vi "S4GUI_002.vi"(7 "Tab ObsEng":enum32{"Obs", "CCD modes", "Eng"}(tab)) -> ()   [LabVIEW 2018] (continued)
            n4169 = call-dynamic "Write Cooler ON_OFF.vi"("error in (no error)"=w9735, "Cooler ON/OFF"=w9727, "Interface in"=w9736) -> ("error out"=w9739:errorcluster, "Interface out"=w9741:refnum<class "Interface.lvclass">)  [unwired: 7 in]
            n4170 = call-dynamic "Write Interface.vi"("error in (no error)"=w9739, "Interface.lvclass"=w9741, "Channel in"=w9743) -> ("error out"=w9738:errorcluster, "Channel out"=w9742:refnum<class "Channel.lvclass">)  [unwired: 7 in]
            n4171 = call-dynamic "Read State Machine.vi"("error in (no error)"=w9738, "Device in"=w9742) -> ("error out"=w9754:errorcluster, "State Machine.lvclass"=w9755:refnum<class "State Machine.lvclass">, "Device out"=w9751:refnum<class "Channel.lvclass">)  [unwired: 7 in]
            n4172 = call "Next State.vi"("error in (no error)"=w9754, "New_State"=u32 30, "State Machine in"=w9755) -> ("error out"=w9749:errorcluster, "State Machine out"=w9752:refnum<class "State Machine.lvclass">)  [unwired: 7 in]
            n4173 = call-dynamic "Write State Machine.vi"("error in (no error)"=w9749, "State Machine.lvclass"=w9752, "Device in"=w9751) -> ("error out"=w9745:errorcluster, "Device out"=w9737:refnum<class "Channel.lvclass">)  [unwired: 7 in]
            n4174 = call-dynamic "Write Channel.vi"("error in (no error)"=w9745, "Channel.lvclass"=w9737, "Acquisition in"=w9750) -> ("error out"=w9746:errorcluster, "Acquisition out"=w9748:refnum<class "Acquisition.lvclass">)  [unwired: 7 in]
            n4175 = call-dynamic "Write AcquisitionA.vi"("error in (no error)"=w9746, "Acquisition.lvclass"=w9748, "S4ACS_GUI in"=w9747) -> ("error out"=w9759:errorcluster, "S4ACS_GUI out"=w9758:refnum<class "S4GUI.lvclass">)  [unwired: 7 in]
          }
        }
      }
      event "cooler ON 2": Value Change {
        n4176 = event-data() -> ("NewVal"=w9760:bool)  [unwired: 1 in]
        n4177 = case shown="True" w9760 {
          tunnel: [w9765 w9800] -> w9764
          tunnel: [w9766 w9799] -> w9763
          tunnel: w9762 -> [w9766 w9770]
          tunnel: w9761 -> [w9765 w9769]
          frame False {
          }
          frame True {
            w9768 = i16 1 items=["Cooler OFF", "Cooler ON"] ("Cooler ON/OFF")
            n4178 = Concatenate Strings("SET COOLER " ("User Event"), "ON ", "CLICKED - CH2" ("User Event")) -> (w9772:string)
            n4179 = call-dynamic "Write User Event.vi"("error in (no error)"=w9769, "User Event"=w9772, "S4GUI in"=w9770) -> ("error out"=w9773:errorcluster, "S4GUI out"=w9775:refnum<class "S4GUI.lvclass">)  [unwired: 7 in]
            n4180 = call "Read AcquisitionB.vi"("error in (no error)"=w9773, "S4ACS_GUI in"=w9775) -> ("error out"=w9797:errorcluster, "Acquisition.lvclass"=w9798:refnum<class "Acquisition.lvclass">, "S4ACS_GUI out"=w9788:refnum<class "S4GUI.lvclass">)  [unwired: 7 in]
            n4181 = call-dynamic "Read Channel.vi"("error in (no error)"=w9797, "Acquisition in"=w9798) -> ("error out"=w9781:errorcluster, "Channel.lvclass"=w9785:refnum<class "Channel.lvclass">, "Acquisition out"=w9791:refnum<class "Acquisition.lvclass">)  [unwired: 7 in]
            n4182 = call-dynamic "Read Interface.vi"("error in (no error)"=w9781, "Channel in"=w9785) -> ("error out"=w9776:errorcluster, "Interface.lvclass"=w9777:refnum<class "Interface.lvclass">, "Channel out"=w9784:refnum<class "Channel.lvclass">)  [unwired: 7 in]
            n4183 = call-dynamic "Write Cooler ON_OFF.vi"("error in (no error)"=w9776, "Cooler ON/OFF"=w9768, "Interface in"=w9777) -> ("error out"=w9780:errorcluster, "Interface out"=w9782:refnum<class "Interface.lvclass">)  [unwired: 7 in]
            n4184 = call-dynamic "Write Interface.vi"("error in (no error)"=w9780, "Interface.lvclass"=w9782, "Channel in"=w9784) -> ("error out"=w9779:errorcluster, "Channel out"=w9783:refnum<class "Channel.lvclass">)  [unwired: 7 in]
            n4185 = call-dynamic "Read State Machine.vi"("error in (no error)"=w9779, "Device in"=w9783) -> ("error out"=w9795:errorcluster, "State Machine.lvclass"=w9796:refnum<class "State Machine.lvclass">, "Device out"=w9792:refnum<class "Channel.lvclass">)  [unwired: 7 in]
            n4186 = call "Next State.vi"("error in (no error)"=w9795, "New_State"=u32 30, "State Machine in"=w9796) -> ("error out"=w9790:errorcluster, "State Machine out"=w9793:refnum<class "State Machine.lvclass">)  [unwired: 7 in]
            n4187 = call-dynamic "Write State Machine.vi"("error in (no error)"=w9790, "State Machine.lvclass"=w9793, "Device in"=w9792) -> ("error out"=w9786:errorcluster, "Device out"=w9778:refnum<class "Channel.lvclass">)  [unwired: 7 in]
            n4188 = call-dynamic "Write Channel.vi"("error in (no error)"=w9786, "Channel.lvclass"=w9778, "Acquisition in"=w9791) -> ("error out"=w9787:errorcluster, "Acquisition out"=w9789:refnum<class "Acquisition.lvclass">)  [unwired: 7 in]
            n4189 = call "Write AcquisitionB.vi"("error in (no error)"=w9787, "Acquisition.lvclass"=w9789, "S4ACS_GUI in"=w9788) -> ("error out"=w9800:errorcluster, "S4ACS_GUI out"=w9799:refnum<class "S4GUI.lvclass">)  [unwired: 7 in]
          }
        }
      }
      event "cooler ON 3": Value Change {
        n4190 = event-data() -> ("NewVal"=w9801:bool)  [unwired: 1 in]
        n4191 = case shown="True" w9801 {
          tunnel: [w9806 w9841] -> w9805
          tunnel: [w9807 w9840] -> w9804
          tunnel: w9803 -> [w9807 w9811]
          tunnel: w9802 -> [w9806 w9810]
          frame False {
          }
          frame True {
            w9809 = i16 1 items=["Cooler OFF", "Cooler ON"] ("Cooler ON/OFF")
            n4192 = Concatenate Strings("SET COOLER " ("User Event"), "ON ", "CLICKED - CH3" ("User Event")) -> (w9813:string)
            n4193 = call-dynamic "Write User Event.vi"("error in (no error)"=w9810, "User Event"=w9813, "S4GUI in"=w9811) -> ("error out"=w9814:errorcluster, "S4GUI out"=w9816:refnum<class "S4GUI.lvclass">)  [unwired: 7 in]
            n4194 = call-dynamic "Read AcquisitionC.vi"("error in (no error)"=w9814, "S4ACS_GUI in"=w9816) -> ("error out"=w9838:errorcluster, "Acquisition.lvclass"=w9839:refnum<class "Acquisition.lvclass">, "S4ACS_GUI out"=w9829:refnum<class "S4GUI.lvclass">)  [unwired: 7 in]
            n4195 = call-dynamic "Read Channel.vi"("error in (no error)"=w9838, "Acquisition in"=w9839) -> ("error out"=w9822:errorcluster, "Channel.lvclass"=w9826:refnum<class "Channel.lvclass">, "Acquisition out"=w9832:refnum<class "Acquisition.lvclass">)  [unwired: 7 in]
            n4196 = call-dynamic "Read Interface.vi"("error in (no error)"=w9822, "Channel in"=w9826) -> ("error out"=w9817:errorcluster, "Interface.lvclass"=w9818:refnum<class "Interface.lvclass">, "Channel out"=w9825:refnum<class "Channel.lvclass">)  [unwired: 7 in]
            n4197 = call-dynamic "Write Cooler ON_OFF.vi"("error in (no error)"=w9817, "Cooler ON/OFF"=w9809, "Interface in"=w9818) -> ("error out"=w9821:errorcluster, "Interface out"=w9823:refnum<class "Interface.lvclass">)  [unwired: 7 in]
            n4198 = call-dynamic "Write Interface.vi"("error in (no error)"=w9821, "Interface.lvclass"=w9823, "Channel in"=w9825) -> ("error out"=w9820:errorcluster, "Channel out"=w9824:refnum<class "Channel.lvclass">)  [unwired: 7 in]
            n4199 = call-dynamic "Read State Machine.vi"("error in (no error)"=w9820, "Device in"=w9824) -> ("error out"=w9836:errorcluster, "State Machine.lvclass"=w9837:refnum<class "State Machine.lvclass">, "Device out"=w9833:refnum<class "Channel.lvclass">)  [unwired: 7 in]
            n4200 = call "Next State.vi"("error in (no error)"=w9836, "New_State"=u32 30, "State Machine in"=w9837) -> ("error out"=w9831:errorcluster, "State Machine out"=w9834:refnum<class "State Machine.lvclass">)  [unwired: 7 in]
            n4201 = call-dynamic "Write State Machine.vi"("error in (no error)"=w9831, "State Machine.lvclass"=w9834, "Device in"=w9833) -> ("error out"=w9827:errorcluster, "Device out"=w9819:refnum<class "Channel.lvclass">)  [unwired: 7 in]
            n4202 = call-dynamic "Write Channel.vi"("error in (no error)"=w9827, "Channel.lvclass"=w9819, "Acquisition in"=w9832) -> ("error out"=w9828:errorcluster, "Acquisition out"=w9830:refnum<class "Acquisition.lvclass">)  [unwired: 7 in]
            n4203 = call-dynamic "Write AcquisitionC.vi"("error in (no error)"=w9828, "Acquisition.lvclass"=w9830, "S4ACS_GUI in"=w9829) -> ("error out"=w9841:errorcluster, "S4ACS_GUI out"=w9840:refnum<class "S4GUI.lvclass">)  [unwired: 7 in]
          }
        }
      }
      event "cooler ON 4": Value Change {
        n4204 = event-data() -> ("NewVal"=w9842:bool)  [unwired: 1 in]
        n4205 = case shown="True" w9842 {
          tunnel: [w9847 w9882] -> w9846
          tunnel: [w9848 w9881] -> w9845
          tunnel: w9844 -> [w9848 w9852]
          tunnel: w9843 -> [w9847 w9851]
          frame False {
          }
          frame True {
            w9850 = i16 1 items=["Cooler OFF", "Cooler ON"] ("Cooler ON/OFF")
            n4206 = Concatenate Strings("SET COOLER " ("User Event"), "ON ", "CLICKED - CH4" ("User Event")) -> (w9854:string)
            n4207 = call-dynamic "Write User Event.vi"("error in (no error)"=w9851, "User Event"=w9854, "S4GUI in"=w9852) -> ("error out"=w9855:errorcluster, "S4GUI out"=w9857:refnum<class "S4GUI.lvclass">)  [unwired: 7 in]
            n4208 = call-dynamic "Read AcquisitionD.vi"("error in (no error)"=w9855, "S4ACS_GUI in"=w9857) -> ("error out"=w9879:errorcluster, "Acquisition.lvclass"=w9880:refnum<class "Acquisition.lvclass">, "S4ACS_GUI out"=w9870:refnum<class "S4GUI.lvclass">)  [unwired: 7 in]
            n4209 = call-dynamic "Read Channel.vi"("error in (no error)"=w9879, "Acquisition in"=w9880) -> ("error out"=w9863:errorcluster, "Channel.lvclass"=w9867:refnum<class "Channel.lvclass">, "Acquisition out"=w9873:refnum<class "Acquisition.lvclass">)  [unwired: 7 in]
            n4210 = call-dynamic "Read Interface.vi"("error in (no error)"=w9863, "Channel in"=w9867) -> ("error out"=w9858:errorcluster, "Interface.lvclass"=w9859:refnum<class "Interface.lvclass">, "Channel out"=w9866:refnum<class "Channel.lvclass">)  [unwired: 7 in]
            n4211 = call-dynamic "Write Cooler ON_OFF.vi"("error in (no error)"=w9858, "Cooler ON/OFF"=w9850, "Interface in"=w9859) -> ("error out"=w9862:errorcluster, "Interface out"=w9864:refnum<class "Interface.lvclass">)  [unwired: 7 in]
            n4212 = call-dynamic "Write Interface.vi"("error in (no error)"=w9862, "Interface.lvclass"=w9864, "Channel in"=w9866) -> ("error out"=w9861:errorcluster, "Channel out"=w9865:refnum<class "Channel.lvclass">)  [unwired: 7 in]
            n4213 = call-dynamic "Read State Machine.vi"("error in (no error)"=w9861, "Device in"=w9865) -> ("error out"=w9877:errorcluster, "State Machine.lvclass"=w9878:refnum<class "State Machine.lvclass">, "Device out"=w9874:refnum<class "Channel.lvclass">)  [unwired: 7 in]
            n4214 = call "Next State.vi"("error in (no error)"=w9877, "New_State"=u32 30, "State Machine in"=w9878) -> ("error out"=w9872:errorcluster, "State Machine out"=w9875:refnum<class "State Machine.lvclass">)  [unwired: 7 in]
            n4215 = call-dynamic "Write State Machine.vi"("error in (no error)"=w9872, "State Machine.lvclass"=w9875, "Device in"=w9874) -> ("error out"=w9868:errorcluster, "Device out"=w9860:refnum<class "Channel.lvclass">)  [unwired: 7 in]
            n4216 = call-dynamic "Write Channel.vi"("error in (no error)"=w9868, "Channel.lvclass"=w9860, "Acquisition in"=w9873) -> ("error out"=w9869:errorcluster, "Acquisition out"=w9871:refnum<class "Acquisition.lvclass">)  [unwired: 7 in]
            n4217 = call-dynamic "Write AcquisitionD.vi"("error in (no error)"=w9869, "Acquisition.lvclass"=w9871, "S4ACS_GUI in"=w9870) -> ("error out"=w9882:errorcluster, "S4ACS_GUI out"=w9881:refnum<class "S4GUI.lvclass">)  [unwired: 7 in]
          }
        }
      }
      event "cooler OFF 1": Value Change {
        n4218 = event-data() -> ("NewVal"=w9883:bool)  [unwired: 1 in]
        n4219 = case shown="True" w9883 {
          tunnel: [w9888 w9923] -> w9887
          tunnel: [w9889 w9922] -> w9886
          tunnel: w9885 -> [w9889 w9893]
          tunnel: w9884 -> [w9888 w9892]
          frame False {
          }
          frame True {
            w9891 = i16 0 items=["Cooler OFF", "Cooler ON"] ("Cooler ON/OFF")
            n4220 = Concatenate Strings("SET COOLER " ("User Event"), "OFF ", "CLICKED - CH1" ("User Event")) -> (w9895:string)
            n4221 = call-dynamic "Write User Event.vi"("error in (no error)"=w9892, "User Event"=w9895, "S4GUI in"=w9893) -> ("error out"=w9896:errorcluster, "S4GUI out"=w9898:refnum<class "S4GUI.lvclass">)  [unwired: 7 in]
            n4222 = call-dynamic "Read AcquisitionA.vi"("error in (no error)"=w9896, "S4ACS_GUI in"=w9898) -> ("error out"=w9920:errorcluster, "Acquisition.lvclass"=w9921:refnum<class "Acquisition.lvclass">, "S4ACS_GUI out"=w9911:refnum<class "S4GUI.lvclass">)  [unwired: 7 in]
            n4223 = call-dynamic "Read Channel.vi"("error in (no error)"=w9920, "Acquisition in"=w9921) -> ("error out"=w9904:errorcluster, "Channel.lvclass"=w9908:refnum<class "Channel.lvclass">, "Acquisition out"=w9914:refnum<class "Acquisition.lvclass">)  [unwired: 7 in]
            n4224 = call-dynamic "Read Interface.vi"("error in (no error)"=w9904, "Channel in"=w9908) -> ("error out"=w9899:errorcluster, "Interface.lvclass"=w9900:refnum<class "Interface.lvclass">, "Channel out"=w9907:refnum<class "Channel.lvclass">)  [unwired: 7 in]
            n4225 = call-dynamic "Write Cooler ON_OFF.vi"("error in (no error)"=w9899, "Cooler ON/OFF"=w9891, "Interface in"=w9900) -> ("error out"=w9903:errorcluster, "Interface out"=w9905:refnum<class "Interface.lvclass">)  [unwired: 7 in]
            n4226 = call-dynamic "Write Interface.vi"("error in (no error)"=w9903, "Interface.lvclass"=w9905, "Channel in"=w9907) -> ("error out"=w9902:errorcluster, "Channel out"=w9906:refnum<class "Channel.lvclass">)  [unwired: 7 in]
            n4227 = call-dynamic "Read State Machine.vi"("error in (no error)"=w9902, "Device in"=w9906) -> ("error out"=w9918:errorcluster, "State Machine.lvclass"=w9919:refnum<class "State Machine.lvclass">, "Device out"=w9915:refnum<class "Channel.lvclass">)  [unwired: 7 in]
            n4228 = call "Next State.vi"("error in (no error)"=w9918, "New_State"=u32 30, "State Machine in"=w9919) -> ("error out"=w9913:errorcluster, "State Machine out"=w9916:refnum<class "State Machine.lvclass">)  [unwired: 7 in]
            n4229 = call-dynamic "Write State Machine.vi"("error in (no error)"=w9913, "State Machine.lvclass"=w9916, "Device in"=w9915) -> ("error out"=w9909:errorcluster, "Device out"=w9901:refnum<class "Channel.lvclass">)  [unwired: 7 in]
            n4230 = call-dynamic "Write Channel.vi"("error in (no error)"=w9909, "Channel.lvclass"=w9901, "Acquisition in"=w9914) -> ("error out"=w9910:errorcluster, "Acquisition out"=w9912:refnum<class "Acquisition.lvclass">)  [unwired: 7 in]
            n4231 = call-dynamic "Write AcquisitionA.vi"("error in (no error)"=w9910, "Acquisition.lvclass"=w9912, "S4ACS_GUI in"=w9911) -> ("error out"=w9923:errorcluster, "S4ACS_GUI out"=w9922:refnum<class "S4GUI.lvclass">)  [unwired: 7 in]
          }
        }
      }
      event "cooler OFF 2": Value Change {
        n4232 = event-data() -> ("NewVal"=w9924:bool)  [unwired: 1 in]
        n4233 = case shown="True" w9924 {
          tunnel: [w9929 w9964] -> w9928
          tunnel: [w9930 w9963] -> w9927
          tunnel: w9926 -> [w9930 w9934]
          tunnel: w9925 -> [w9929 w9933]
          frame False {
          }
          frame True {
            w9932 = i16 0 items=["Cooler OFF", "Cooler ON"] ("Cooler ON/OFF")
            n4234 = Concatenate Strings("SET COOLER " ("User Event"), "OFF ", "CLICKED - CH2" ("User Event")) -> (w9936:string)
            n4235 = call-dynamic "Write User Event.vi"("error in (no error)"=w9933, "User Event"=w9936, "S4GUI in"=w9934) -> ("error out"=w9937:errorcluster, "S4GUI out"=w9939:refnum<class "S4GUI.lvclass">)  [unwired: 7 in]
            n4236 = call "Read AcquisitionB.vi"("error in (no error)"=w9937, "S4ACS_GUI in"=w9939) -> ("error out"=w9961:errorcluster, "Acquisition.lvclass"=w9962:refnum<class "Acquisition.lvclass">, "S4ACS_GUI out"=w9952:refnum<class "S4GUI.lvclass">)  [unwired: 7 in]
            n4237 = call-dynamic "Read Channel.vi"("error in (no error)"=w9961, "Acquisition in"=w9962) -> ("error out"=w9945:errorcluster, "Channel.lvclass"=w9949:refnum<class "Channel.lvclass">, "Acquisition out"=w9955:refnum<class "Acquisition.lvclass">)  [unwired: 7 in]
            n4238 = call-dynamic "Read Interface.vi"("error in (no error)"=w9945, "Channel in"=w9949) -> ("error out"=w9940:errorcluster, "Interface.lvclass"=w9941:refnum<class "Interface.lvclass">, "Channel out"=w9948:refnum<class "Channel.lvclass">)  [unwired: 7 in]
            n4239 = call-dynamic "Write Cooler ON_OFF.vi"("error in (no error)"=w9940, "Cooler ON/OFF"=w9932, "Interface in"=w9941) -> ("error out"=w9944:errorcluster, "Interface out"=w9946:refnum<class "Interface.lvclass">)  [unwired: 7 in]
            n4240 = call-dynamic "Write Interface.vi"("error in (no error)"=w9944, "Interface.lvclass"=w9946, "Channel in"=w9948) -> ("error out"=w9943:errorcluster, "Channel out"=w9947:refnum<class "Channel.lvclass">)  [unwired: 7 in]
            n4241 = call-dynamic "Read State Machine.vi"("error in (no error)"=w9943, "Device in"=w9947) -> ("error out"=w9959:errorcluster, "State Machine.lvclass"=w9960:refnum<class "State Machine.lvclass">, "Device out"=w9956:refnum<class "Channel.lvclass">)  [unwired: 7 in]
            n4242 = call "Next State.vi"("error in (no error)"=w9959, "New_State"=u32 30, "State Machine in"=w9960) -> ("error out"=w9954:errorcluster, "State Machine out"=w9957:refnum<class "State Machine.lvclass">)  [unwired: 7 in]
            n4243 = call-dynamic "Write State Machine.vi"("error in (no error)"=w9954, "State Machine.lvclass"=w9957, "Device in"=w9956) -> ("error out"=w9950:errorcluster, "Device out"=w9942:refnum<class "Channel.lvclass">)  [unwired: 7 in]
            n4244 = call-dynamic "Write Channel.vi"("error in (no error)"=w9950, "Channel.lvclass"=w9942, "Acquisition in"=w9955) -> ("error out"=w9951:errorcluster, "Acquisition out"=w9953:refnum<class "Acquisition.lvclass">)  [unwired: 7 in]
            n4245 = call "Write AcquisitionB.vi"("error in (no error)"=w9951, "Acquisition.lvclass"=w9953, "S4ACS_GUI in"=w9952) -> ("error out"=w9964:errorcluster, "S4ACS_GUI out"=w9963:refnum<class "S4GUI.lvclass">)  [unwired: 7 in]
          }
        }
      }
      event "cooler OFF 3": Value Change {
        n4246 = event-data() -> ("NewVal"=w9965:bool)  [unwired: 1 in]
        n4247 = case shown="True" w9965 {
          tunnel: [w9970 w10005] -> w9969
          tunnel: [w9971 w10004] -> w9968
          tunnel: w9967 -> [w9971 w9975]
          tunnel: w9966 -> [w9970 w9974]
          frame False {
          }
          frame True {
            w9973 = i16 0 items=["Cooler OFF", "Cooler ON"] ("Cooler ON/OFF")
            n4248 = Concatenate Strings("SET COOLER " ("User Event"), "OFF ", "CLICKED - CH3" ("User Event")) -> (w9977:string)
            n4249 = call-dynamic "Write User Event.vi"("error in (no error)"=w9974, "User Event"=w9977, "S4GUI in"=w9975) -> ("error out"=w9978:errorcluster, "S4GUI out"=w9980:refnum<class "S4GUI.lvclass">)  [unwired: 7 in]
            n4250 = call-dynamic "Read AcquisitionC.vi"("error in (no error)"=w9978, "S4ACS_GUI in"=w9980) -> ("error out"=w10002:errorcluster, "Acquisition.lvclass"=w10003:refnum<class "Acquisition.lvclass">, "S4ACS_GUI out"=w9993:refnum<class "S4GUI.lvclass">)  [unwired: 7 in]
            n4251 = call-dynamic "Read Channel.vi"("error in (no error)"=w10002, "Acquisition in"=w10003) -> ("error out"=w9986:errorcluster, "Channel.lvclass"=w9990:refnum<class "Channel.lvclass">, "Acquisition out"=w9996:refnum<class "Acquisition.lvclass">)  [unwired: 7 in]
            n4252 = call-dynamic "Read Interface.vi"("error in (no error)"=w9986, "Channel in"=w9990) -> ("error out"=w9981:errorcluster, "Interface.lvclass"=w9982:refnum<class "Interface.lvclass">, "Channel out"=w9989:refnum<class "Channel.lvclass">)  [unwired: 7 in]
            n4253 = call-dynamic "Write Cooler ON_OFF.vi"("error in (no error)"=w9981, "Cooler ON/OFF"=w9973, "Interface in"=w9982) -> ("error out"=w9985:errorcluster, "Interface out"=w9987:refnum<class "Interface.lvclass">)  [unwired: 7 in]
            n4254 = call-dynamic "Write Interface.vi"("error in (no error)"=w9985, "Interface.lvclass"=w9987, "Channel in"=w9989) -> ("error out"=w9984:errorcluster, "Channel out"=w9988:refnum<class "Channel.lvclass">)  [unwired: 7 in]
            n4255 = call-dynamic "Read State Machine.vi"("error in (no error)"=w9984, "Device in"=w9988) -> ("error out"=w10000:errorcluster, "State Machine.lvclass"=w10001:refnum<class "State Machine.lvclass">, "Device out"=w9997:refnum<class "Channel.lvclass">)  [unwired: 7 in]
            n4256 = call "Next State.vi"("error in (no error)"=w10000, "New_State"=u32 30, "State Machine in"=w10001) -> ("error out"=w9995:errorcluster, "State Machine out"=w9998:refnum<class "State Machine.lvclass">)  [unwired: 7 in]
            n4257 = call-dynamic "Write State Machine.vi"("error in (no error)"=w9995, "State Machine.lvclass"=w9998, "Device in"=w9997) -> ("error out"=w9991:errorcluster, "Device out"=w9983:refnum<class "Channel.lvclass">)  [unwired: 7 in]
            n4258 = call-dynamic "Write Channel.vi"("error in (no error)"=w9991, "Channel.lvclass"=w9983, "Acquisition in"=w9996) -> ("error out"=w9992:errorcluster, "Acquisition out"=w9994:refnum<class "Acquisition.lvclass">)  [unwired: 7 in]
            n4259 = call-dynamic "Write AcquisitionC.vi"("error in (no error)"=w9992, "Acquisition.lvclass"=w9994, "S4ACS_GUI in"=w9993) -> ("error out"=w10005:errorcluster, "S4ACS_GUI out"=w10004:refnum<class "S4GUI.lvclass">)  [unwired: 7 in]
          }
        }
      }
      event "cooler OFF 4": Value Change {
        n4260 = event-data() -> ("NewVal"=w10006:bool)  [unwired: 1 in]
        n4261 = case shown="True" w10006 {
          tunnel: [w10011 w10046] -> w10010
          tunnel: [w10012 w10045] -> w10009
          tunnel: w10008 -> [w10012 w10016]
          tunnel: w10007 -> [w10011 w10015]
          frame False {
          }
          frame True {
            w10014 = i16 0 items=["Cooler OFF", "Cooler ON"] ("Cooler ON/OFF")
            n4262 = Concatenate Strings("SET COOLER " ("User Event"), "OFF ", "CLICKED - CH4" ("User Event")) -> (w10018:string)
            n4263 = call-dynamic "Write User Event.vi"("error in (no error)"=w10015, "User Event"=w10018, "S4GUI in"=w10016) -> ("error out"=w10019:errorcluster, "S4GUI out"=w10021:refnum<class "S4GUI.lvclass">)  [unwired: 7 in]
            n4264 = call-dynamic "Read AcquisitionD.vi"("error in (no error)"=w10019, "S4ACS_GUI in"=w10021) -> ("error out"=w10043:errorcluster, "Acquisition.lvclass"=w10044:refnum<class "Acquisition.lvclass">, "S4ACS_GUI out"=w10034:refnum<class "S4GUI.lvclass">)  [unwired: 7 in]
            n4265 = call-dynamic "Read Channel.vi"("error in (no error)"=w10043, "Acquisition in"=w10044) -> ("error out"=w10027:errorcluster, "Channel.lvclass"=w10031:refnum<class "Channel.lvclass">, "Acquisition out"=w10037:refnum<class "Acquisition.lvclass">)  [unwired: 7 in]
            n4266 = call-dynamic "Read Interface.vi"("error in (no error)"=w10027, "Channel in"=w10031) -> ("error out"=w10022:errorcluster, "Interface.lvclass"=w10023:refnum<class "Interface.lvclass">, "Channel out"=w10030:refnum<class "Channel.lvclass">)  [unwired: 7 in]
            n4267 = call-dynamic "Write Cooler ON_OFF.vi"("error in (no error)"=w10022, "Cooler ON/OFF"=w10014, "Interface in"=w10023) -> ("error out"=w10026:errorcluster, "Interface out"=w10028:refnum<class "Interface.lvclass">)  [unwired: 7 in]
            n4268 = call-dynamic "Write Interface.vi"("error in (no error)"=w10026, "Interface.lvclass"=w10028, "Channel in"=w10030) -> ("error out"=w10025:errorcluster, "Channel out"=w10029:refnum<class "Channel.lvclass">)  [unwired: 7 in]
            n4269 = call-dynamic "Read State Machine.vi"("error in (no error)"=w10025, "Device in"=w10029) -> ("error out"=w10041:errorcluster, "State Machine.lvclass"=w10042:refnum<class "State Machine.lvclass">, "Device out"=w10038:refnum<class "Channel.lvclass">)  [unwired: 7 in]
            n4270 = call "Next State.vi"("error in (no error)"=w10041, "New_State"=u32 30, "State Machine in"=w10042) -> ("error out"=w10036:errorcluster, "State Machine out"=w10039:refnum<class "State Machine.lvclass">)  [unwired: 7 in]
            n4271 = call-dynamic "Write State Machine.vi"("error in (no error)"=w10036, "State Machine.lvclass"=w10039, "Device in"=w10038) -> ("error out"=w10032:errorcluster, "Device out"=w10024:refnum<class "Channel.lvclass">)  [unwired: 7 in]
            n4272 = call-dynamic "Write Channel.vi"("error in (no error)"=w10032, "Channel.lvclass"=w10024, "Acquisition in"=w10037) -> ("error out"=w10033:errorcluster, "Acquisition out"=w10035:refnum<class "Acquisition.lvclass">)  [unwired: 7 in]
            n4273 = call-dynamic "Write AcquisitionD.vi"("error in (no error)"=w10033, "Acquisition.lvclass"=w10035, "S4ACS_GUI in"=w10034) -> ("error out"=w10046:errorcluster, "S4ACS_GUI out"=w10045:refnum<class "S4GUI.lvclass">)  [unwired: 7 in]
          }
        }
      }
      event "Set Temp 1": Value Change {
        n4274 = event-data() -> ("NewVal"=w10047:bool)  [unwired: 1 in]
        n4275 = case shown="True" w10047 {
          tunnel: w10051 -> [w10053 w10070]
          tunnel: w10050 -> [w10052 w10069]
          tunnel: [w10052 w10059] -> w10049
          tunnel: [w10053 w10060] -> w10048
          frame False {
          }
          frame True {
            # "Carrega a maior temperatura\nentre target atual e o target do controle."
            # "Carrega o valor da temperatura target de acordo com a conf CCD"
            n4276 = call-dynamic "Read AcquisitionA.vi"("error in (no error)"=w10069, "S4ACS_GUI in"=w10070) -> ("error out"=w10072:errorcluster, "Acquisition.lvclass"=w10071:refnum<class "Acquisition.lvclass">, "S4ACS_GUI out"=w10056:refnum<class "S4GUI.lvclass">)  [unwired: 7 in]
            n4277 = call-dynamic "Read Channel.vi"("error in (no error)"=w10072, "Acquisition in"=w10071) -> ("error out"=w10083:errorcluster, "Channel.lvclass"=w10082:refnum<class "Channel.lvclass">, "Acquisition out"=w10055:refnum<class "Acquisition.lvclass">)  [unwired: 7 in]
            n4278 = call-dynamic "ValidateConfig.vi"("error in (no error)"=w10083, "Channel in"=w10082) -> ("error out"=w10089:errorcluster, "Channel out"=w10088:refnum<class "Channel.lvclass">)  [unwired: 7 in, 1 out]
            n4279 = call-dynamic "Read Interface.vi"("error in (no error)"=w10089, "Channel in"=w10088) -> ("error out"=w10085:errorcluster, "Interface.lvclass"=w10084:refnum<class "Interface.lvclass">, "Channel out"=w10078:refnum<class "Channel.lvclass">)  [unwired: 7 in]
            n4280 = call-dynamic "Read Temperature.vi"("error in (no error)"=w10085, "Interface in"=w10084) -> ("error out"=w10086:errorcluster, "Temperature"=w10090:i8, "Interface out"=w10087:refnum<class "Interface.lvclass">)  [unwired: 7 in]
            n4281 = Greater?(x=w10090, y="Target Temp 1") -> (0:w10058:bool)
            n4282 = Select(t=w10090, s=w10058, f="Target Temp 1") -> (s? t:f=w10063:i8)
            n4283 = call-dynamic "Write Temperature.vi"("error in (no error)"=w10086, "Temperature"=w10063, "Interface in"=w10087) -> ("error out"=w10080:errorcluster, "Interface out"=w10077:refnum<class "Interface.lvclass">)  [unwired: 7 in]
            n4284 = call-dynamic "Write Interface.vi"("error in (no error)"=w10080, "Interface.lvclass"=w10077, "Channel in"=w10078) -> ("error out"=w10081:errorcluster, "Channel out"=w10079:refnum<class "Channel.lvclass">)  [unwired: 7 in]
            n4285 = case shown="True" w10058 {
              tunnel: w10081 -> [w10115 w10118]
              tunnel: w10079 -> [w10114 w10125]
              tunnel: [w10113 w10125] -> w10076
              tunnel: [w10112 w10124] -> w10075
              tunnel: w10056 -> [w10092 w10120]
              tunnel: [w10092 w10123] -> w10057
              tunnel: w10055 -> [w10091 w10122]
              tunnel: [w10091 w10121] -> w10054
              frame False {
                # "input ok"
                n4286 = call-dynamic "Read State Machine.vi"("error in (no error)"=w10115, "Device in"=w10114) -> ("error out"=w10094:errorcluster, "State Machine.lvclass"=w10101:refnum<class "State Machine.lvclass">, "Device out"=w10110:refnum<class "Channel.lvclass">)  [unwired: 7 in]
                n4287 = call-dynamic "Read ref StatesQueue.vi"("error in (no error)"=w10094, "State Machine in"=w10101) -> ("error out"=w10104:errorcluster, "ref StatesQueue"=w10098:refnum<queue>, "State Machine out"=w10100:refnum<class "State Machine.lvclass">)  [unwired: 7 in]
                n4288 = Flush Queue(queue=w10098, error in (no error)=w10104) -> (queue out=w10097:refnum<queue>, error out=w10106:errorcluster)  [unwired: 1 out]
                n4289 = Enqueue Element(queue=w10097, element=u32 35 ("State"), error in (no error)=w10106) -> (queue out=w10096:refnum<queue>, error out=w10107:errorcluster)  [unwired: 1 in, 1 out]
                n4290 = Enqueue Element(queue=w10096, element=u32 37 ("State"), error in (no error)=w10107) -> (queue out=w10095:refnum<queue>, error out=w10105:errorcluster)  [unwired: 1 in, 1 out]
                n4291 = call-dynamic "Write ref StatesQueue.vi"("error in (no error)"=w10105, "ref StatesQueue"=w10095, "State Machine in"=w10100) -> ("error out"=w10093:errorcluster, "State Machine out"=w10099:refnum<class "State Machine.lvclass">)  [unwired: 7 in]
                n4292 = call "Next State.vi"("error in (no error)"=w10093, "New_State"=u32 0, "State Machine in"=w10099) -> ("error out"=w10111:errorcluster, "State Machine out"=w10109:refnum<class "State Machine.lvclass">)  [unwired: 7 in]
                n4293 = call-dynamic "Write State Machine.vi"("error in (no error)"=w10111, "State Machine.lvclass"=w10109, "Device in"=w10110) -> ("error out"=w10112:errorcluster, "Device out"=w10113:refnum<class "Channel.lvclass">)  [unwired: 7 in]
              }
              frame True {
                # "input error"
                n4294 = call-dynamic "Read SET temp error mode.vi"("error in (no error)"=w10118, "S4GUI in"=w10120) -> ("error out"=w10117:errorcluster, "SET temp error mode"=w10116:bool, "S4GUI out"=w10119:refnum<class "S4GUI.lvclass">)  [unwired: 7 in]
                n4295 = case shown="False" w10116 {
                  tunnel: [w10134 w10149] -> w10124
                  tunnel: [w10133 w10148] -> w10123
                  tunnel: w10119 -> [w10132 w10148]
                  tunnel: w10117 -> [w10129 w10150]
                  tunnel: w10122 -> [w10127 w10147]
                  tunnel: [w10126 w10147] -> w10121
                  frame False {
                    # "last error msg"
                    n4296 = call-dynamic "Read sync.vi"("error in (no error)"=w10129, "S4ACS_GUI in"=w10132) -> ("error out"=w10128:errorcluster, "sync"=w10130:bool, "S4ACS_GUI out"=w10131:refnum<class "S4GUI.lvclass">)  [unwired: 7 in]
                    n4297 = case shown="False" w10130 {
                      tunnel: w10128 -> [w10137 w10146]
                      tunnel: [w10136 w10145] -> w10134
                      tunnel: [w10140 w10144] -> w10133
                      tunnel: w10131 -> [w10140 w10142]
                      tunnel: w10127 -> [w10138 w10141]
                      tunnel: [w10135 w10141] -> w10126
                      frame False {
                        n4298 = call-dynamic "Write Acq_state.vi"("error in (no error)"=w10137, "Acq_state"=u32 240, "Acquisition in"=w10138) -> ("error out"=w10136:errorcluster, "Acquisition out"=w10135:refnum<class "Acquisition.lvclass">)  [unwired: 7 in]
                      }
                      frame True {
                        n4299 = call-dynamic "Write Obs_state.vi"("error in (no error)"=w10146, "Obs_state"=u32 240, "S4ACS_GUI in"=w10142) -> ("error out"=w10145:errorcluster, "S4ACS_GUI out"=w10144:refnum<class "S4GUI.lvclass">)  [unwired: 7 in]
                      }
                    }
                  }
                  frame True {
                    # "popup msg"
                    n4300 = disable-structure shown="Enabled" {
                      disable-tunnel: w10150 -> [w10152 w10159]
                      disable-tunnel: [w10151 w10159] -> w10149
                      frame Enabled {
                        w10154 = FALSE ("Wait Until Done")
                        n4301 = call <vilib>:"Application Directory.vi"() -> ("Application Directory"=w10158:path)
                        n4302 = Build Path(base path=w10158, name or relative path="MsgSetTemp.vi") -> (appended path=w10155:path)
                        n4303 = Open VI Reference(vi path=w10155, error in (no error)=w10152) -> (vi reference=w10156:refnum<vi>, error out=w10157:errorcluster)  [unwired: 4 in]
                        n4304 = invoke class="VI" method="Run VI"(reference=w10156, error in=w10157, "Wait until done"=w10154, "Auto Dispose Ref"=w10154) -> (error out=w10151:errorcluster)  [unwired: 1 in, 4 out]
                      }
                      frame Disabled {
                        n4305 = One Button Dialog(message="ERROR: Invalid input value. It must be \nequal or greater than the minimum for \nthe current CCD setup.", button name ("OK")="OK" ("T button name (\"OK\")")) -> ()  [unwired: 1 out]
                      }
                    }
                  }
                }
              }
            }
            n4306 = Number To Decimal String(number="Target Temp 1") -> (decimal integer string=w10062:string)  [unwired: 1 in]
            n4307 = call-dynamic "Write Channel.vi"("error in (no error)"=w10075, "Channel.lvclass"=w10076, "Acquisition in"=w10054) -> ("error out"=w10074:errorcluster, "Acquisition out"=w10073:refnum<class "Acquisition.lvclass">)  [unwired: 7 in]
            n4308 = Concatenate Strings("SET TEMP [" ("User Event"), w10062, "] CLICKED - CH1" ("User Event")) -> (w10068:string)
            n4309 = call-dynamic "Write AcquisitionA.vi"("error in (no error)"=w10074, "Acquisition.lvclass"=w10073, "S4ACS_GUI in"=w10057) -> ("error out"=w10064:errorcluster, "S4ACS_GUI out"=w10065:refnum<class "S4GUI.lvclass">)  [unwired: 7 in]
            n4310 = call-dynamic "Write User Event.vi"("error in (no error)"=w10064, "User Event"=w10068, "S4GUI in"=w10065) -> ("error out"=w10059:errorcluster, "S4GUI out"=w10060:refnum<class "S4GUI.lvclass">)  [unwired: 7 in]
          }
        }
      }
      event "Set Temp 2": Value Change {
        n4311 = event-data() -> ("NewVal"=w10162:bool)  [unwired: 1 in]
        n4312 = case shown="True" w10162 {
          tunnel: w10166 -> [w10168 w10188]
          tunnel: w10165 -> [w10167 w10187]
          tunnel: [w10167 w10180] -> w10164
          tunnel: [w10168 w10182] -> w10163
          frame False {
          }
          frame True {
            # "Carrega a maior temperatura\nentre target atual e o target do controle."
            # "Carrega o valor da temperatura target de acordo com a conf CCD"
            n4313 = call "Read AcquisitionB.vi"("error in (no error)"=w10187, "S4ACS_GUI in"=w10188) -> ("error out"=w10204:errorcluster, "Acquisition.lvclass"=w10205:refnum<class "Acquisition.lvclass">, "S4ACS_GUI out"=w10175:refnum<class "S4GUI.lvclass">)  [unwired: 7 in]
            n4314 = call-dynamic "Read Channel.vi"("error in (no error)"=w10204, "Acquisition in"=w10205) -> ("error out"=w10197:errorcluster, "Channel.lvclass"=w10198:refnum<class "Channel.lvclass">, "Acquisition out"=w10176:refnum<class "Acquisition.lvclass">)  [unwired: 7 in]
            n4315 = call-dynamic "ValidateConfig.vi"("error in (no error)"=w10197, "Channel in"=w10198) -> ("error out"=w10191:errorcluster, "Channel out"=w10192:refnum<class "Channel.lvclass">)  [unwired: 7 in, 1 out]
            n4316 = call-dynamic "Read Interface.vi"("error in (no error)"=w10191, "Channel in"=w10192) -> ("error out"=w10195:errorcluster, "Interface.lvclass"=w10196:refnum<class "Interface.lvclass">, "Channel out"=w10200:refnum<class "Channel.lvclass">)  [unwired: 7 in]
            n4317 = call-dynamic "Read Temperature.vi"("error in (no error)"=w10195, "Interface in"=w10196) -> ("error out"=w10194:errorcluster, "Temperature"=w10190:i8, "Interface out"=w10193:refnum<class "Interface.lvclass">)  [unwired: 7 in]
            n4318 = Greater?(x=w10190, y="Target Temp 2") -> (0:w10173:bool)
            n4319 = Select(t=w10190, s=w10173, f="Target Temp 2") -> (s? t:f=w10189:i32)
            n4320 = call-dynamic "Write Temperature.vi"("error in (no error)"=w10194, "Temperature"=w10189, "Interface in"=w10193) -> ("error out"=w10199:errorcluster, "Interface out"=w10201:refnum<class "Interface.lvclass">)  [unwired: 7 in]
            n4321 = call-dynamic "Write Interface.vi"("error in (no error)"=w10199, "Interface.lvclass"=w10201, "Channel in"=w10200) -> ("error out"=w10174:errorcluster, "Channel out"=w10177:refnum<class "Channel.lvclass">)  [unwired: 7 in]
            n4322 = case shown="True" w10173 {
              tunnel: w10174 -> [w10230 w10235]
              tunnel: w10177 -> [w10229 w10237]
              tunnel: [w10228 w10237] -> w10170
              tunnel: [w10227 w10240] -> w10169
              tunnel: w10175 -> [w10207 w10236]
              tunnel: [w10207 w10239] -> w10172
              tunnel: w10176 -> [w10206 w10231]
              tunnel: [w10206 w10238] -> w10171
              frame False {
                # "input ok"
                n4323 = call-dynamic "Read State Machine.vi"("error in (no error)"=w10230, "Device in"=w10229) -> ("error out"=w10209:errorcluster, "State Machine.lvclass"=w10216:refnum<class "State Machine.lvclass">, "Device out"=w10225:refnum<class "Channel.lvclass">)  [unwired: 7 in]
                n4324 = call-dynamic "Read ref StatesQueue.vi"("error in (no error)"=w10209, "State Machine in"=w10216) -> ("error out"=w10219:errorcluster, "ref StatesQueue"=w10213:refnum<queue>, "State Machine out"=w10215:refnum<class "State Machine.lvclass">)  [unwired: 7 in]
                n4325 = Flush Queue(queue=w10213, error in (no error)=w10219) -> (queue out=w10212:refnum<queue>, error out=w10221:errorcluster)  [unwired: 1 out]
                n4326 = Enqueue Element(queue=w10212, element=u32 35 ("State"), error in (no error)=w10221) -> (queue out=w10211:refnum<queue>, error out=w10222:errorcluster)  [unwired: 1 in, 1 out]
                n4327 = Enqueue Element(queue=w10211, element=u32 37 ("State"), error in (no error)=w10222) -> (queue out=w10210:refnum<queue>, error out=w10220:errorcluster)  [unwired: 1 in, 1 out]
                n4328 = call-dynamic "Write ref StatesQueue.vi"("error in (no error)"=w10220, "ref StatesQueue"=w10210, "State Machine in"=w10215) -> ("error out"=w10208:errorcluster, "State Machine out"=w10214:refnum<class "State Machine.lvclass">)  [unwired: 7 in]
                n4329 = call "Next State.vi"("error in (no error)"=w10208, "New_State"=u32 0, "State Machine in"=w10214) -> ("error out"=w10226:errorcluster, "State Machine out"=w10224:refnum<class "State Machine.lvclass">)  [unwired: 7 in]
                n4330 = call-dynamic "Write State Machine.vi"("error in (no error)"=w10226, "State Machine.lvclass"=w10224, "Device in"=w10225) -> ("error out"=w10227:errorcluster, "Device out"=w10228:refnum<class "Channel.lvclass">)  [unwired: 7 in]
              }
              frame True {
                # "input error"
                n4331 = call-dynamic "Read SET temp error mode.vi"("error in (no error)"=w10235, "S4GUI in"=w10236) -> ("error out"=w10232:errorcluster, "SET temp error mode"=w10234:bool, "S4GUI out"=w10233:refnum<class "S4GUI.lvclass">)  [unwired: 7 in]
                n4332 = case shown="False" w10234 {
                  tunnel: [w10249 w10262] -> w10240
                  tunnel: [w10248 w10271] -> w10239
                  tunnel: [w10244 w10270] -> w10238
                  tunnel: w10231 -> [w10243 w10270]
                  tunnel: w10233 -> [w10242 w10271]
                  tunnel: w10232 -> [w10241 w10263]
                  frame False {
                    # "last error msg"
                    n4333 = call-dynamic "Read sync.vi"("error in (no error)"=w10241, "S4ACS_GUI in"=w10242) -> ("error out"=w10245:errorcluster, "sync"=w10246:bool, "S4ACS_GUI out"=w10247:refnum<class "S4GUI.lvclass">)  [unwired: 7 in]
                    n4334 = case shown="True" w10246 {
                      tunnel: w10245 -> [w10252 w10261]
                      tunnel: [w10251 w10260] -> w10249
                      tunnel: [w10255 w10259] -> w10248
                      tunnel: w10247 -> [w10255 w10257]
                      tunnel: w10243 -> [w10253 w10256]
                      tunnel: [w10250 w10256] -> w10244
                      frame False {
                        n4335 = call-dynamic "Write Acq_state.vi"("error in (no error)"=w10252, "Acq_state"=u32 240, "Acquisition in"=w10253) -> ("error out"=w10251:errorcluster, "Acquisition out"=w10250:refnum<class "Acquisition.lvclass">)  [unwired: 7 in]
                      }
                      frame True {
                        n4336 = call-dynamic "Write Obs_state.vi"("error in (no error)"=w10261, "Obs_state"=u32 240, "S4ACS_GUI in"=w10257) -> ("error out"=w10260:errorcluster, "S4ACS_GUI out"=w10259:refnum<class "S4GUI.lvclass">)  [unwired: 7 in]
                      }
                    }
                  }
                  frame True {
                    w10265 = FALSE ("Wait Until Done")
                    # "popup msg"
                    n4337 = call <vilib>:"Application Directory.vi"() -> ("Application Directory"=w10269:path)
                    n4338 = Build Path(base path=w10269, name or relative path="MsgSetTemp.vi") -> (appended path=w10266:path)
                    n4339 = Open VI Reference(vi path=w10266, error in (no error)=w10263) -> (vi reference=w10267:refnum<vi>, error out=w10268:errorcluster)  [unwired: 4 in]
                    n4340 = invoke class="VI" method="Run VI"(reference=w10267, error in=w10268, "Wait until done"=w10265, "Auto Dispose Ref"=w10265) -> (error out=w10262:errorcluster)  [unwired: 1 in, 4 out]
                  }
                }
              }
            }
            n4341 = Number To Decimal String(number="Target Temp 2") -> (decimal integer string=w10178:string)  [unwired: 1 in]
            n4342 = call-dynamic "Write Channel.vi"("error in (no error)"=w10169, "Channel.lvclass"=w10170, "Acquisition in"=w10171) -> ("error out"=w10202:errorcluster, "Acquisition out"=w10203:refnum<class "Acquisition.lvclass">)  [unwired: 7 in]
            n4343 = Concatenate Strings("SET TEMP [" ("User Event"), w10178, "] CLICKED - CH2" ("User Event")) -> (w10186:string)
            n4344 = call "Write AcquisitionB.vi"("error in (no error)"=w10202, "Acquisition.lvclass"=w10203, "S4ACS_GUI in"=w10172) -> ("error out"=w10181:errorcluster, "S4ACS_GUI out"=w10183:refnum<class "S4GUI.lvclass">)  [unwired: 7 in]
            n4345 = call-dynamic "Write User Event.vi"("error in (no error)"=w10181, "User Event"=w10186, "S4GUI in"=w10183) -> ("error out"=w10180:errorcluster, "S4GUI out"=w10182:refnum<class "S4GUI.lvclass">)  [unwired: 7 in]
          }
        }
      }
      event "Set Temp 3": Value Change {
        n4346 = event-data() -> ("NewVal"=w10272:bool)  [unwired: 1 in]
        n4347 = case shown="True" w10272 {
          tunnel: w10276 -> [w10278 w10298]
          tunnel: w10275 -> [w10277 w10297]
          tunnel: [w10277 w10289] -> w10274
          tunnel: [w10278 w10291] -> w10273
          frame False {
          }
          frame True {
            # "Carrega a maior temperatura\nentre target atual e o target do controle."
            # "Carrega o valor da temperatura target de acordo com a conf CCD"
            n4348 = call-dynamic "Read AcquisitionC.vi"("error in (no error)"=w10297, "S4ACS_GUI in"=w10298) -> ("error out"=w10300:errorcluster, "Acquisition.lvclass"=w10299:refnum<class "Acquisition.lvclass">, "S4ACS_GUI out"=w10280:refnum<class "S4GUI.lvclass">)  [unwired: 7 in]
            n4349 = call-dynamic "Read Channel.vi"("error in (no error)"=w10300, "Acquisition in"=w10299) -> ("error out"=w10307:errorcluster, "Channel.lvclass"=w10306:refnum<class "Channel.lvclass">, "Acquisition out"=w10281:refnum<class "Acquisition.lvclass">)  [unwired: 7 in]
            n4350 = call-dynamic "ValidateConfig.vi"("error in (no error)"=w10307, "Channel in"=w10306) -> ("error out"=w10313:errorcluster, "Channel out"=w10312:refnum<class "Channel.lvclass">)  [unwired: 7 in, 1 out]
            n4351 = call-dynamic "Read Interface.vi"("error in (no error)"=w10313, "Channel in"=w10312) -> ("error out"=w10309:errorcluster, "Interface.lvclass"=w10308:refnum<class "Interface.lvclass">, "Channel out"=w10304:refnum<class "Channel.lvclass">)  [unwired: 7 in]
            n4352 = call-dynamic "Read Temperature.vi"("error in (no error)"=w10309, "Interface in"=w10308) -> ("error out"=w10310:errorcluster, "Temperature"=w10314:i8, "Interface out"=w10311:refnum<class "Interface.lvclass">)  [unwired: 7 in]
            n4353 = Greater?(x=w10314, y="Target Temp 3") -> (0:w10279:bool)
            n4354 = Select(t=w10314, s=w10279, f="Target Temp 3") -> (s? t:f=w10315:i32)
            n4355 = call-dynamic "Write Temperature.vi"("error in (no error)"=w10310, "Temperature"=w10315, "Interface in"=w10311) -> ("error out"=w10305:errorcluster, "Interface out"=w10303:refnum<class "Interface.lvclass">)  [unwired: 7 in]
            n4356 = call-dynamic "Write Interface.vi"("error in (no error)"=w10305, "Interface.lvclass"=w10303, "Channel in"=w10304) -> ("error out"=w10282:errorcluster, "Channel out"=w10287:refnum<class "Channel.lvclass">)  [unwired: 7 in]
            n4357 = case shown="True" w10279 {
              tunnel: w10282 -> [w10340 w10341]
              tunnel: w10287 -> [w10339 w10347]
              tunnel: [w10338 w10347] -> w10286
              tunnel: [w10337 w10350] -> w10283
              tunnel: w10280 -> [w10317 w10346]
              tunnel: [w10317 w10349] -> w10284
              tunnel: w10281 -> [w10316 w10344]
              tunnel: [w10316 w10348] -> w10285
              frame False {
                # "input ok"
                n4358 = call-dynamic "Read State Machine.vi"("error in (no error)"=w10340, "Device in"=w10339) -> ("error out"=w10319:errorcluster, "State Machine.lvclass"=w10326:refnum<class "State Machine.lvclass">, "Device out"=w10335:refnum<class "Channel.lvclass">)  [unwired: 7 in]
                n4359 = call-dynamic "Read ref StatesQueue.vi"("error in (no error)"=w10319, "State Machine in"=w10326) -> ("error out"=w10329:errorcluster, "ref StatesQueue"=w10323:refnum<queue>, "State Machine out"=w10325:refnum<class "State Machine.lvclass">)  [unwired: 7 in]
                n4360 = Flush Queue(queue=w10323, error in (no error)=w10329) -> (queue out=w10322:refnum<queue>, error out=w10331:errorcluster)  [unwired: 1 out]
                n4361 = Enqueue Element(queue=w10322, element=u32 35 ("State"), error in (no error)=w10331) -> (queue out=w10321:refnum<queue>, error out=w10332:errorcluster)  [unwired: 1 in, 1 out]
                n4362 = Enqueue Element(queue=w10321, element=u32 37 ("State"), error in (no error)=w10332) -> (queue out=w10320:refnum<queue>, error out=w10330:errorcluster)  [unwired: 1 in, 1 out]
                n4363 = call-dynamic "Write ref StatesQueue.vi"("error in (no error)"=w10330, "ref StatesQueue"=w10320, "State Machine in"=w10325) -> ("error out"=w10318:errorcluster, "State Machine out"=w10324:refnum<class "State Machine.lvclass">)  [unwired: 7 in]
                n4364 = call "Next State.vi"("error in (no error)"=w10318, "New_State"=u32 0, "State Machine in"=w10324) -> ("error out"=w10336:errorcluster, "State Machine out"=w10334:refnum<class "State Machine.lvclass">)  [unwired: 7 in]
                n4365 = call-dynamic "Write State Machine.vi"("error in (no error)"=w10336, "State Machine.lvclass"=w10334, "Device in"=w10335) -> ("error out"=w10337:errorcluster, "Device out"=w10338:refnum<class "Channel.lvclass">)  [unwired: 7 in]
              }
              frame True {
                # "input error"
                n4366 = call-dynamic "Read SET temp error mode.vi"("error in (no error)"=w10341, "S4GUI in"=w10346) -> ("error out"=w10342:errorcluster, "SET temp error mode"=w10343:bool, "S4GUI out"=w10345:refnum<class "S4GUI.lvclass">)  [unwired: 7 in]
                n4367 = case shown="False" w10343 {
                  tunnel: [w10359 w10372] -> w10350
                  tunnel: [w10358 w10381] -> w10349
                  tunnel: w10345 -> [w10357 w10381]
                  tunnel: w10342 -> [w10354 w10373]
                  tunnel: w10344 -> [w10352 w10380]
                  tunnel: [w10351 w10380] -> w10348
                  frame False {
                    # "last error msg"
                    n4368 = call-dynamic "Read sync.vi"("error in (no error)"=w10354, "S4ACS_GUI in"=w10357) -> ("error out"=w10353:errorcluster, "sync"=w10355:bool, "S4ACS_GUI out"=w10356:refnum<class "S4GUI.lvclass">)  [unwired: 7 in]
                    n4369 = case shown="True" w10355 {
                      tunnel: w10353 -> [w10362 w10371]
                      tunnel: [w10361 w10370] -> w10359
                      tunnel: [w10365 w10369] -> w10358
                      tunnel: w10356 -> [w10365 w10367]
                      tunnel: w10352 -> [w10363 w10366]
                      tunnel: [w10360 w10366] -> w10351
                      frame False {
                        n4370 = call-dynamic "Write Acq_state.vi"("error in (no error)"=w10362, "Acq_state"=u32 240, "Acquisition in"=w10363) -> ("error out"=w10361:errorcluster, "Acquisition out"=w10360:refnum<class "Acquisition.lvclass">)  [unwired: 7 in]
                      }
                      frame True {
                        n4371 = call-dynamic "Write Obs_state.vi"("error in (no error)"=w10371, "Obs_state"=u32 240, "S4ACS_GUI in"=w10367) -> ("error out"=w10370:errorcluster, "S4ACS_GUI out"=w10369:refnum<class "S4GUI.lvclass">)  [unwired: 7 in]
                      }
                    }
                  }
                  frame True {
                    w10375 = FALSE ("Wait Until Done")
                    # "popup msg"
                    n4372 = call <vilib>:"Application Directory.vi"() -> ("Application Directory"=w10376:path)
                    n4373 = Build Path(base path=w10376, name or relative path="MsgSetTemp.vi") -> (appended path=w10379:path)
                    n4374 = Open VI Reference(vi path=w10379, error in (no error)=w10373) -> (vi reference=w10378:refnum<vi>, error out=w10377:errorcluster)  [unwired: 4 in]
                    n4375 = invoke class="VI" method="Run VI"(reference=w10378, error in=w10377, "Wait until done"=w10375, "Auto Dispose Ref"=w10375) -> (error out=w10372:errorcluster)  [unwired: 1 in, 4 out]
                  }
                }
              }
            }
            n4376 = Number To Decimal String(number="Target Temp 3") -> (decimal integer string=w10293:string)  [unwired: 1 in]
            n4377 = call-dynamic "Write Channel.vi"("error in (no error)"=w10283, "Channel.lvclass"=w10286, "Acquisition in"=w10285) -> ("error out"=w10302:errorcluster, "Acquisition out"=w10301:refnum<class "Acquisition.lvclass">)  [unwired: 7 in]
            n4378 = call-dynamic "Write AcquisitionC.vi"("error in (no error)"=w10302, "Acquisition.lvclass"=w10301, "S4ACS_GUI in"=w10284) -> ("error out"=w10290:errorcluster, "S4ACS_GUI out"=w10292:refnum<class "S4GUI.lvclass">)  [unwired: 7 in]
            n4379 = Concatenate Strings("SET TEMP [" ("User Event"), w10293, "] CLICKED - CH3" ("User Event")) -> (w10296:string)
            n4380 = call-dynamic "Write User Event.vi"("error in (no error)"=w10290, "User Event"=w10296, "S4GUI in"=w10292) -> ("error out"=w10289:errorcluster, "S4GUI out"=w10291:refnum<class "S4GUI.lvclass">)  [unwired: 7 in]
          }
        }
      }
      event "Set Temp 4": Value Change {
        n4381 = event-data() -> ("NewVal"=w10382:bool)  [unwired: 1 in]
        n4382 = case shown="True" w10382 {
